vi "createRetValueVI.vi"(4 "visitor class path":path, 6 "visitor base path":path, 8 "error in (no error)":errorcluster, 10 "Indicators":cluster{"Style":u32, "Label.Text":string, i32}[](array[cluster]), 11 "Class Name":string) -> (0 "error out":errorcluster)   [LabVIEW 2009, in "HGF_VisitorGenerator.lvlib"]
doc: "create visitor member VI to read return values (=outputs of public interface VI)"
uses:
  HGF_VisitorGenerator.lvlib
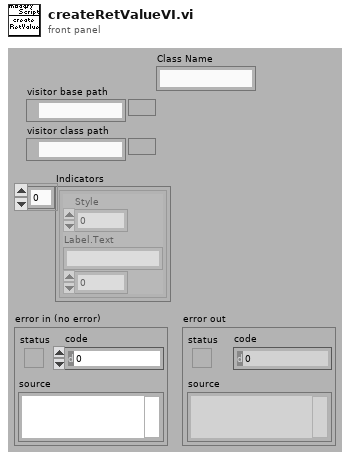
[diagram p1: front panel]
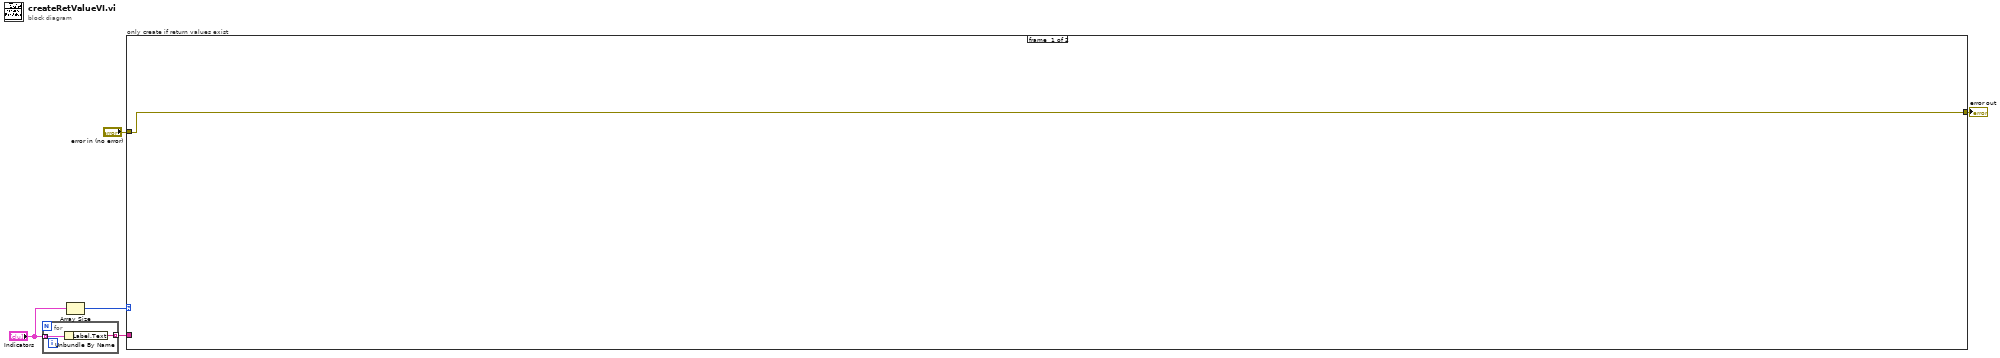
[diagram p0: block diagram]
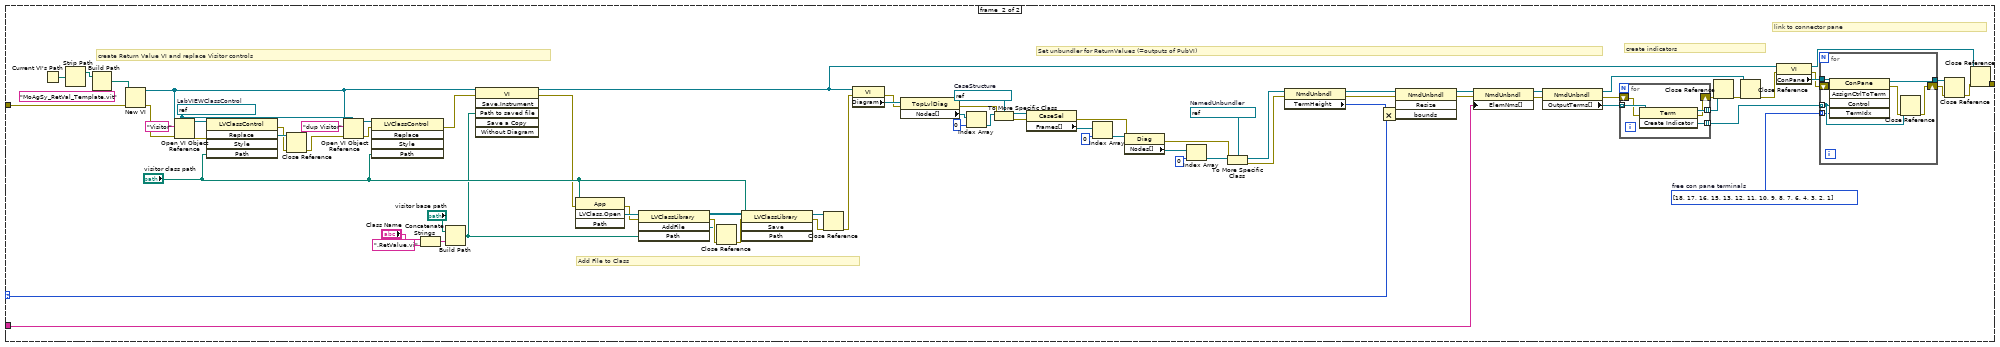
[diagram p2: hidden frame]
diagram:
  n1 = for {
    tunnel: "Indicators" -> [w7] mode=indexing
    tunnel: [w6] -> w5 mode=indexing
    n2 = Unbundle By Name(w7) -> ("Label.Text"=w6:string)
  }
  n3 = Array Size(array="Indicators") -> (size(s)=w1:i32)
  n4 = case "only create if return values exist" shown="Default" w1 {
    selector: w1 -> [_ w12]
    tunnel: w5 -> [_ w58]
    tunnel: [w8 w41] -> w3
    tunnel: "error in (no error)" -> [w8 w13]
    frame #0 {
    }
    frame #1 {
      w24 = refnum<vi> refnum  # CaseStructure
      w40 = u32[] [18, 17, 16, 15, 13, 12, 11, 10, 9, 8, 7, 6, 4, 3, 2, 1]  # free con pane terminals
      w16 = refnum<vi> refnum  # NamedUnbundler
      w80 = refnum<vi> refnum  # LabVIEWClassControl
      # "create indicators"
      # "link to connector pane"
      # "Set unbundler for ReturnValues (=outputs of PubVI)"
      # "create Return Value VI and replace Visitor controls"
      # "Add File to Class"
      n5 = Current VI's Path() -> (path=w88:path)
      n6 = Strip Path(path=w88) -> (stripped path=w9:path)  [unwired: 1 out]
      n7 = Build Path(base path=w9, name or relative path="MoAgSy_RetVal_Template.vit") -> (appended path=w11:path)
      n8 = New VI(8:w13, 10:w11) -> (0:w32:errorcluster, 3:w75:refnum<vi>)  [unwired: 5 in]
      n9 = Open VI Object Reference(7:w80, 8:w32, 10:"Visitor" ("name/order"), 11:w75) -> (0:w85:errorcluster, 3:w86:refnum<vi>)
      n10 = invoke class="LVClassControl" method="Replace"(reference=w86, error in=w85, "Path"="visitor class path") -> (error out=w83:errorcluster, "Replace"=w84:refnum<vi>)  [unwired: 2 in, 3 out]
      n11 = Close Reference(reference=w84, error in (no error)=w83) -> (error out=w81:errorcluster)
      n12 = Open VI Object Reference(7:w80, 8:w81, 10:"dup Visitor" ("name/order"), 11:w75) -> (0:w78:errorcluster, 3:w79:refnum<vi>)
      n13 = invoke class="LVClassControl" method="Replace"(reference=w79, error in=w78, "Path"="visitor class path") -> (error out=w74:errorcluster)  [unwired: 2 in, 4 out]
      n14 = Concatenate Strings("Class Name", ".RetValue.vi" ("string")) -> (w70:string)
      n15 = Build Path(base path="visitor base path", name or relative path=w70) -> (appended path=w69:path)
      n16 = invoke class="VI" method="Save.Instrument"(reference=w75, error in=w74, "Path to saved file"=w69) -> (reference out=w36:refnum<vi>, error out=w68:errorcluster)  [unwired: 3 in, 4 out]
      n17 = invoke class="App" method="LVClass.Open"(error in=w68, "Path"="visitor class path") -> (error out=w67:errorcluster, "LVClass.Open"=w89:refnum<vi>)  [unwired: 2 in, 2 out]
      n18 = invoke class="LVClassLibrary" method="AddFile"(reference=w89, error in=w67, "Path"=w69) -> (reference out=w77:refnum<vi>, error out=w39:errorcluster, "AddFile"=w38:refnum<vi>)  [unwired: 1 in, 1 out]
      n19 = Close Reference(reference=w38, error in (no error)=w39) -> (error out=w37:errorcluster)
      n20 = invoke class="LVClassLibrary" method="Save"(reference=w77, error in=w37, "Path"="visitor class path") -> (reference out=w65:refnum<vi>, error out=w66:errorcluster)  [unwired: 1 in, 2 out]
      n21 = Close Reference(reference=w65, error in (no error)=w66) -> (error out=w33:errorcluster)
      n22 = property class="VI"(reference=w36, error in=w33) -> (error out=w34:errorcluster, "Diagram"=w35:refnum<vi>)  [unwired: 1 out]
      n23 = property class="TopLvlDiag"(reference=w35, error in=w34) -> (error out=w22:errorcluster, "Nodes[]"=w30:refnum<vi>[])  [unwired: 1 out]
      n24 = Index Array(array=w30, index=0) -> (element=w23:refnum<vi>)
      n25 = To More Specific Class(target class=w24, reference=w23, error in=w22) -> (specific class reference=w25:refnum<vi>, error out=w26:errorcluster)
      n26 = property class="CaseSel"(reference=w25, error in=w26) -> (error out=w21:errorcluster, "Frames[]"=w28:refnum<vi>[])  [unwired: 1 out]
      n27 = Index Array(array=w28, index=0) -> (element=w29:refnum<vi>)
      n28 = property class="Diag"(reference=w29, error in=w21) -> (error out=w18:errorcluster, "Nodes[]"=w19:refnum<vi>[])  [unwired: 1 out]
      n29 = Index Array(array=w19, index=0) -> (element=w17:refnum<vi>)
      n30 = To More Specific Class(target class=w16, reference=w17, error in=w18) -> (specific class reference=w15:refnum<vi>, error out=w14:errorcluster)
      n31 = property class="NmdUnbndl"(reference=w15, error in=w14) -> (reference out=w63:refnum<vi>, error out=w64:errorcluster, "TermHeight"=w57:i32)
      n32 = Multiply(x=w57, y=w12) -> (x*y=w56:i32)
      n33 = invoke class="NmdUnbndl" method="Resize"(reference=w63, error in=w64, "bounds"=w56) -> (reference out=w62:refnum<vi>, error out=w61:errorcluster)  [unwired: 1 in, 2 out]
      n34 = property class="NmdUnbndl"(reference=w62, error in=w61, "ElemNms[]"=w58) -> (reference out=w60:refnum<vi>, error out=w59:errorcluster)
      n35 = property class="NmdUnbndl"(reference=w60, error in=w59) -> (reference out=w50:refnum<vi>, error out=w55:errorcluster, "OutputTerms[]"=w54:refnum<vi>[])
      n36 = for {
        shift-right: [w98] -> w53
        shift-left: w55 -> [w100]
        tunnel: w54 -> [w101] mode=indexing
        tunnel: [w99] -> w52 mode=indexing
        tunnel: [w97] -> w47 mode=indexing
        n37 = invoke class="Term" method="Create Indicator"(reference=w101, error in=w100) -> (reference out=w99:refnum<vi>, error out=w98:errorcluster, "Create Indicator"=w97:refnum<vi>)  [unwired: 1 in]
      }
      n38 = Close Reference(reference=w52, error in (no error)=w53) -> (error out=w51:errorcluster)
      n39 = Close Reference(reference=w50, error in (no error)=w51) -> (error out=w49:errorcluster)
      n40 = property class="VI"(reference=w36, error in=w49) -> (reference out=w42:refnum<vi>, error out=w46:errorcluster, "ConPane"=w48:refnum<vi>)
      n41 = for {
        tunnel: w48 -> [w96]
        tunnel: w47 -> [w93] mode=indexing
        tunnel: [w95] -> w44
        shift-right: [w91] -> w45
        shift-left: w46 -> [w94]
        tunnel: w40 -> [w90] mode=indexing
        n42 = invoke class="ConPane" method="AssignCtrlToTerm"(reference=w96, error in=w94, "Control"=w93, "TermIdx"=w90) -> (reference out=w95:refnum<vi>, error out=w92:errorcluster)  [unwired: 1 in, 3 out]
        n43 = Close Reference(reference=w93, error in (no error)=w92) -> (error out=w91:errorcluster)
      }
      n44 = Close Reference(reference=w44, error in (no error)=w45) -> (error out=w43:errorcluster)
      n45 = Close Reference(reference=w42, error in (no error)=w43) -> (error out=w41:errorcluster)
    }
  }
  "error out" <- w3
